vi "Read Camera Attributes.vi"(6 "Read (true)":bool, 8 "error in":errorcluster, 10 "Camera Attributes In":string, 11 "Session In":T1) -> (0 "error out":errorcluster, 2 "Camera Attributes":string, 3 "Session Out":T1)   [LabVIEW 2012]
uses:
  <vilib>/userDefined/High Color/IMAQdx.ctl
  <vilib>/vision/driver/NI_Vision_Acquisition_Software.lvlib
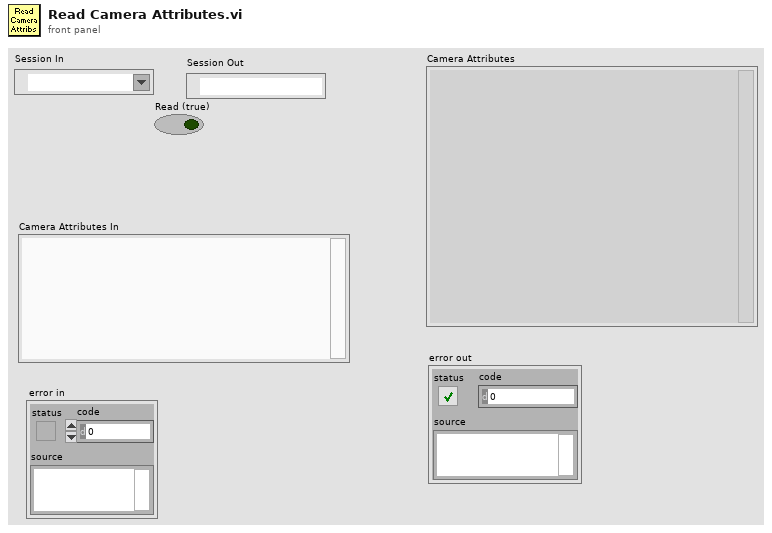
[diagram p1: front panel]
types:
  T1 = typedef "IMAQdx.ctl" = refnum<k21>
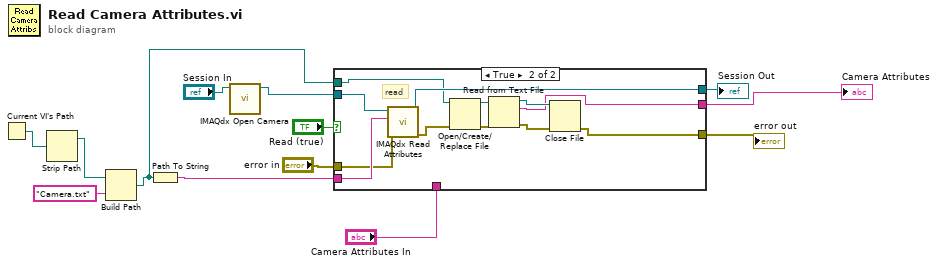
[diagram p0: block diagram]
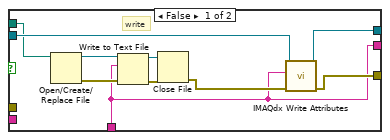
[diagram p2: hidden frame]
diagram:
  n1 = Current VI's Path() -> (path=w13:path)
  n2 = Strip Path(path=w13) -> (stripped path=w12:path)  [unwired: 1 out]
  n3 = Build Path(base path=w12, name or relative path="Camera.txt") -> (appended path=w5:path)
  n4 = Path To String(path=w5) -> (string=w10:string)
  n5 = call <vilib>:"IMAQdx Open Camera.vi"("Session In"="Session In") -> ("Session Out"=w1:T1)  [unwired: 9 in, 1 out]
  n6 = case shown="True" "Read (true)" {
    tunnel: w10 -> [_ w35]
    tunnel: w1 -> [w23 w34]
    tunnel: [w15 w28] -> w6
    tunnel: "error in" -> [_ w33]
    tunnel: [w22 w32] -> w8
    tunnel: w5 -> [w21 w27]
    tunnel: "Camera Attributes In" -> [w14 _]
    tunnel: [w14 w24] -> w3
    frame False {
      # "write"
      n7 = Open/Create/Replace File(file path (use dialog)=w21) -> (refnum out=w19:refnum<file>, error out=w20:errorcluster)  [unwired: 5 in, 1 out]
      n8 = Write to Text File(file (use dialog)=w19, text=w14, error in=w20) -> (refnum out=w18:refnum<file>, error out=w17:errorcluster)  [unwired: 1 in, 1 out]
      n9 = Close File(refnum=w18, error in=w17) -> (error out=w16:errorcluster)  [unwired: 1 out]
      n10 = call <vilib>:"IMAQdx Write Attributes.vi"("error in"=w16, "Filename"=w14, "Session In"=w23) -> ("error out"=w15:errorcluster, "Session Out"=w22:T1)  [unwired: 7 in]
    }
    frame True {
      # "read"
      n11 = call <vilib>:"IMAQdx Read Attributes.vi"("error in"=w33, "Filename"=w35, "Session In"=w34) -> ("error out"=w29:errorcluster, "Session Out"=w32:T1)  [unwired: 7 in]
      n12 = Open/Create/Replace File(file path (use dialog)=w27, error in=w29) -> (refnum out=w26:refnum<file>, error out=w30:errorcluster)  [unwired: 4 in, 1 out]
      n13 = Read from Text File(file (use dialog)=w26, error in=w30) -> (refnum out=w25:refnum<file>, text=w24:string, error out=w31:errorcluster)  [unwired: 2 in, 1 out]
      n14 = Close File(refnum=w25, error in=w31) -> (error out=w28:errorcluster)  [unwired: 1 out]
    }
  }
  "Camera Attributes" <- w3
  "error out" <- w6
  "Session Out" <- w8
